vi "StepName.vi"(8 "error in (no error)":errorcluster, 11 "Sequence Context In":refnum<k7>) -> (0 "error out":errorcluster, 1 "DataSource":string, 2 "Result":string, 3 "Name":string)   [LabVIEW 2021]
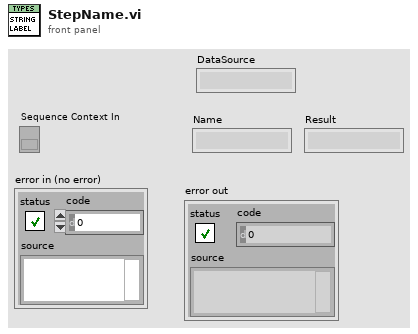
[diagram p1: front panel]
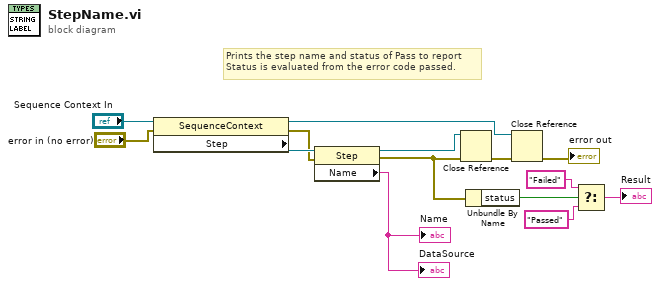
[diagram p0: block diagram]
diagram:
  # "Prints the step name and status of Pass to report\nStatus is evaluated from the error code passed."
  n1 = property class="SequenceContext"(reference="Sequence Context In", error in="error in (no error)") -> (reference out=w6:refnum<k7>, error out=w10:errorcluster, "Step"=w12:refnum<k7>)
  n2 = property class="Step"(reference=w12, error in=w10) -> (reference out=w7:refnum<k7>, error out=w9:errorcluster, "Name"=→"Name" →"DataSource":string)
  n3 = Close Reference(reference=w7, error in (no error)=w9) -> (error out=w8:errorcluster)
  n4 = Unbundle By Name(w9) -> ("status"=w4:bool)
  n5 = Close Reference(reference=w6, error in (no error)=w8) -> (error out=→"error out":errorcluster)
  n6 = Select(t="Failed" ("f"), s=w4, f="Passed") -> (s? t:f=→"Result":string)
